vi "create_new_dataset.vi"(8 "error in (no error)":errorcluster, 9 "Variant":variant, 10 "Path":string, 11 "pcfs_hdf5_log in":refnum<class "pcfs_hdf5_log.lvclass">) -> (0 "error out":errorcluster, 3 "pcfs_hdf5_log out":refnum<class "pcfs_hdf5_log.lvclass">)   [LabVIEW 2015, in "pcfs_hdf5_log.lvclass"]
uses:
  pcfs_hdf5_log.lvclass
  pcfs_hdf5_log.lvclass/pcfs_hdf5_log.ctl
  <vilib>/UPVI/lvhdf5/property.llb/LVH5PClassId.ctl
  <vilib>/UPVI/lvhdf5/dataset.llb/LVH5D Operation.ctl
  Detector_Class/Picoquant/Hydraharp/hydraharp_panel/hpanel_acq_modes.ctl
  <vilib>/UPVI/lvhdf5/library.llb/HDF5 Ref.ctl
  <vilib>/UPVI/lvhdf5/group.llb/OpenCreateGroup (String).vi
  <vilib>/UPVI/lvhdf5/datatype.llb/LVH5Tcreate_dataset_type (Variant).vi
  <vilib>/UPVI/lvhdf5/datatype.llb/LVH5Tcreate_dataset_type.xnode
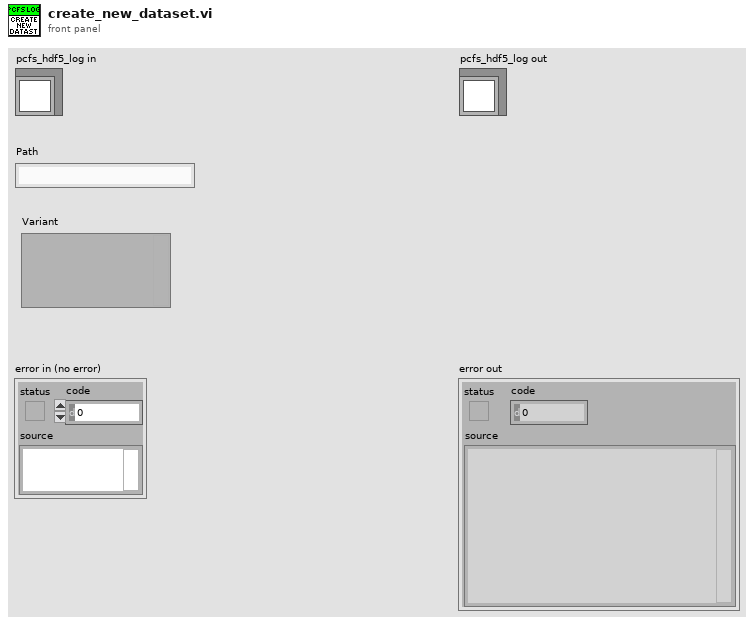
[diagram p1: front panel]
types:
  T1 = typedef "LVH5D Operation.ctl" = enum16{"open", "replace", "create", "open or create", "create or replace", "create or replace with confirmation"}
  T2 = typedef "LVH5PClassId.ctl" = enum32{"H5P_ROOT", "H5P_OBJECT_CREATE", "H5P_FILE_CREATE", "H5P_FILE_ACCESS", "H5P_DATASET_CREATE", "H5P_DATASET_ACCESS", "H5P_DATASET_XFER", "H5P_FILE_MOUNT", "H5P_GROUP_CREATE", "H5P_GROUP_ACCESS", "H5P_DATATYPE_CREATE", "H5P_DATATYPE_ACCESS", "H5P_STRING_CREATE", "H5P_ATTRIBUTE_CREATE", "H5P_OBJECT_COPY", "H5P_LINK_CREATE", "H5P_LINK_ACCESS"}
  T3 = typedef "HDF5 Ref.ctl" = refnum<k1>
  T4 = typedef "hpanel_acq_modes.ctl" = u16
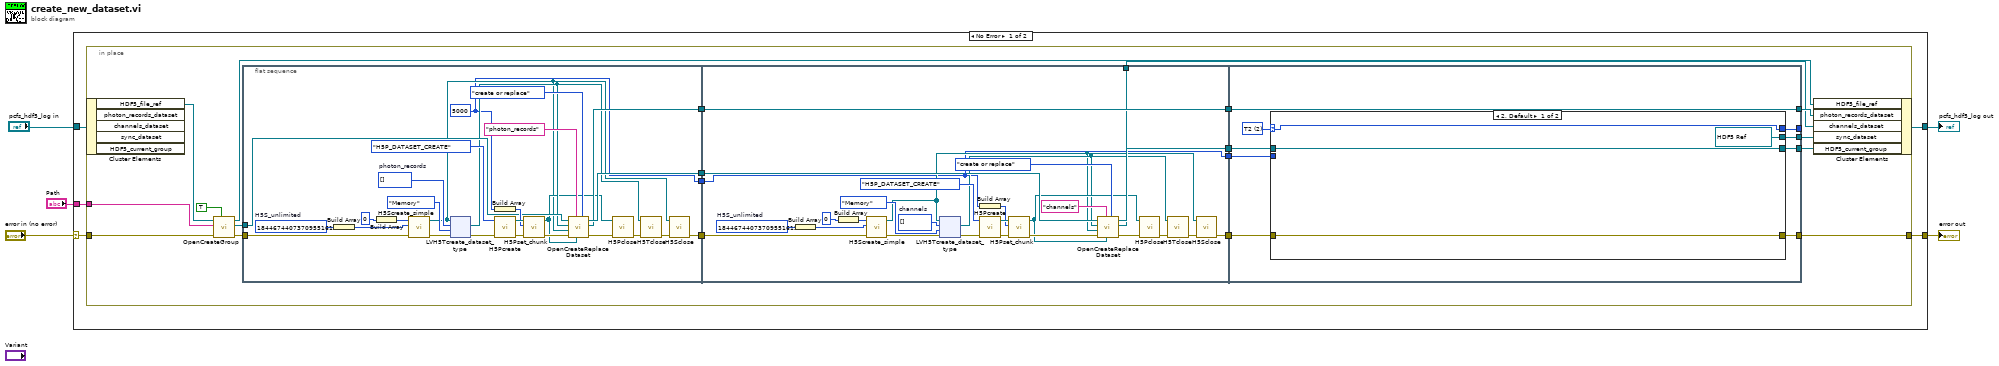
[diagram p0: block diagram]
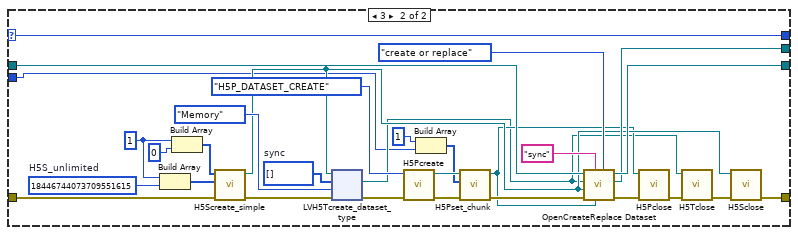
[diagram p2: hidden frame]
diagram:
  n1 = case shown="No Error" "error in (no error)" {
    selector: "error in (no error)" -> [w8 w201]
    tunnel: "pcfs_hdf5_log in" -> [w10 w202]
    tunnel: "Path" -> [w9 _]
    tunnel: [w7 w202] -> w2
    tunnel: [w6 w201] -> w1
    frame No Error {
      n2 = in-place {
        in-place-border: w9 -> [w19]
        in-place-border: w8 -> [w21]
        in-place-border: [w24] -> w6
        n3 = in-place-cluster #1(w10) -> ("HDF5_file_ref"=w17:T3)  [unwired: 4 out]
        n4 = call-poly <vilib>:"OpenCreateGroup.vi"("Create if not found (F)"=TRUE, "error in (no error)"=w21, "Group"=w19, "HDF5 Ref"=w17) -> ("error out"=w20:errorcluster, "HDF5 Group Ref"=w16:T3, "HDF5 Ref out"=w14:T3)  [unwired: 5 in]
        n5 = flat-sequence {
          tunnel: w20 -> [w44]
          tunnel: [w43] -> w29
          tunnel: [w41] -> w28
          tunnel: w16 -> [w40]
          tunnel: [w35] -> w13
          tunnel: [w31] -> w12
          tunnel: w29 -> [w97]
          tunnel: w28 -> [w109]
          tunnel: [w96] -> w27
          tunnel: [w109] -> w26
          tunnel: [w87] -> w25
          tunnel: [w95] -> w23
          tunnel: w13 -> [w98]
          tunnel: w12 -> [w86]
          tunnel: [w86] -> w11
          tunnel: [w142] -> w30
          tunnel: [w138] -> w15
          tunnel: w27 -> [w139]
          tunnel: w26 -> [w142]
          tunnel: w25 -> [w141]
          tunnel: [w140] -> w24
          tunnel: [w137] -> w22
          tunnel: [w136] -> _
          tunnel: w11 -> [w135]
          frame #0 {
            w31 = 5000
            w48 = u64[] []  # photon_records
            w52 = u64 18446744073709551615  # H5S_unlimited
            n6 = Build Array(w52) -> (w51:u64[])
            n7 = Build Array(u64 0 ("element")) -> (w49:u64[])
            n8 = call <vilib>:"H5Screate_simple.vi"("error in (no error)"=w44, "Maximum Dimensions (unlimited)"=w51, "Dimensions"=w49) -> ("error out"=w57:errorcluster, "HDF5 Ref out"=w32:T3)  [unwired: 5 in]
            n9 = xnode "LVH5Tcreate_dataset_type"("HDF5 Location Ref"=w32, "Type"=enum16{"File", "Memory"}."Memory", "error in (no error)"=w57, "Data"=w48) -> ("HDF5 Type Ref"=w34:T3, "error out"=w54:errorcluster)  [unwired: 2 in, 3 out]
            n10 = Build Array(w31) -> (w45:i32[])
            n11 = call <vilib>:"H5Pcreate.vi"("error in (no error)"=w54, "Property List Class"=LVH5PClassId."H5P_DATASET_CREATE") -> ("error out"=w55:errorcluster, "HDF5 Property List Ref"=w56:T3)  [unwired: 6 in]
            n12 = call <vilib>:"H5Pset_chunk.vi"("error in (no error)"=w55, "Dimensions"=w45, "HDF5 Property Ref"=w56) -> ("error out"=w53:errorcluster, "HDF5 Ref out"=w33:T3)  [unwired: 5 in]
            n13 = call <vilib>:"OpenCreateReplace Dataset.vi"("operation (open or create)"=LVH5D_Operation."create or replace", "HDF5 Property List Ref"=w33, "Dataset Path"="photon_records" ("string"), "error in (no error)"=w53, "HDF5 Dataspace Ref"=w32, "HDF5 Datatype Ref"=w34, "HDF5 Ref"=w40) -> ("error out"=w36:errorcluster, "HDF5 Dataset Ref"=w41:T3, "HDF5 Ref out"=w43:T3)  [unwired: 2 in]
            n14 = call <vilib>:"H5Pclose.vi"("error in (no error)"=w36, "HDF5 Property Ref"=w33) -> ("error out"=w38:errorcluster)  [unwired: 7 in]
            n15 = call <vilib>:"H5Tclose.vi"("error in (no error)"=w38, "HDF5 Datatype Ref"=w34) -> ("error out"=w37:errorcluster)  [unwired: 7 in]
            n16 = call <vilib>:"H5Sclose.vi"("error in (no error)"=w37, "HDF5 Dataspace Ref"=w32) -> ("error out"=w35:errorcluster)  [unwired: 7 in]
          }
          frame #1 {
            w85 = u64 18446744073709551615  # H5S_unlimited
            w103 = u8[] []  # channels
            n17 = Build Array(w85) -> (w83:u64[])
            n18 = Build Array(u64 0 ("element")) -> (w82:u64[])
            n19 = call <vilib>:"H5Screate_simple.vi"("error in (no error)"=w98, "Maximum Dimensions (unlimited)"=w83, "Dimensions"=w82) -> ("error out"=w108:errorcluster, "HDF5 Ref out"=w88:T3)  [unwired: 5 in]
            n20 = xnode "LVH5Tcreate_dataset_type"("HDF5 Location Ref"=w88, "Type"=enum16{"File", "Memory"}."Memory", "error in (no error)"=w108, "Data"=w103) -> ("HDF5 Type Ref"=w89:T3, "error out"=w105:errorcluster)  [unwired: 2 in, 3 out]
            n21 = Build Array(w86) -> (w100:i32[])
            n22 = call <vilib>:"H5Pcreate.vi"("error in (no error)"=w105, "Property List Class"=LVH5PClassId."H5P_DATASET_CREATE") -> ("error out"=w106:errorcluster, "HDF5 Property List Ref"=w107:T3)  [unwired: 6 in]
            n23 = call <vilib>:"H5Pset_chunk.vi"("error in (no error)"=w106, "Dimensions"=w100, "HDF5 Property Ref"=w107) -> ("error out"=w104:errorcluster, "HDF5 Ref out"=w90:T3)  [unwired: 5 in]
            n24 = call <vilib>:"OpenCreateReplace Dataset.vi"("operation (open or create)"=LVH5D_Operation."create or replace", "HDF5 Property List Ref"=w90, "Dataset Path"="channels" ("string"), "error in (no error)"=w104, "HDF5 Dataspace Ref"=w88, "HDF5 Datatype Ref"=w89, "HDF5 Ref"=w97) -> ("error out"=w91:errorcluster, "HDF5 Dataset Ref"=w95:T3, "HDF5 Ref out"=w96:T3)  [unwired: 2 in]
            n25 = call <vilib>:"H5Pclose.vi"("error in (no error)"=w91, "HDF5 Property Ref"=w90) -> ("error out"=w93:errorcluster)  [unwired: 7 in]
            n26 = call <vilib>:"H5Tclose.vi"("error in (no error)"=w93, "HDF5 Datatype Ref"=w89) -> ("error out"=w92:errorcluster)  [unwired: 7 in]
            n27 = call <vilib>:"H5Sclose.vi"("error in (no error)"=w92, "HDF5 Dataspace Ref"=w88) -> ("error out"=w87:errorcluster)  [unwired: 7 in]
          }
          frame #2 {
            w134 = T4 2 items=["T2"=2, "T3"=3] ("Mode")
            n28 = case shown="2, Default" w134 {
              selector: w134 -> [w143 w156]
              tunnel: w141 -> [w146 w160]
              tunnel: [w146 w151] -> w140
              tunnel: w139 -> [w145 w159]
              tunnel: [w145 w158] -> w138
              tunnel: [w144 w157] -> w137
              tunnel: [w143 w156] -> w136
              tunnel: w135 -> [_ w147]
              frame 2, Default {
                w144 = T3 refnum items=["HDF5 Ref"] ("HDF5 Dataset Ref")
              }
              frame 3 {
                w166 = u64[] []  # sync
                w169 = u64 1 ("element")
                w171 = u64 18446744073709551615  # H5S_unlimited
                n29 = Build Array(w169, w171) -> (w170:u64[])
                n30 = Build Array(w169, u64 0 ("element")) -> (w167:u64[])
                n31 = call <vilib>:"H5Screate_simple.vi"("error in (no error)"=w160, "Maximum Dimensions (unlimited)"=w170, "Dimensions"=w167) -> ("error out"=w176:errorcluster, "HDF5 Ref out"=w150:T3)  [unwired: 5 in]
                n32 = xnode "LVH5Tcreate_dataset_type"("HDF5 Location Ref"=w150, "Type"=enum16{"File", "Memory"}."Memory", "error in (no error)"=w176, "Data"=w166) -> ("HDF5 Type Ref"=w148:T3, "error out"=w173:errorcluster)  [unwired: 2 in, 3 out]
                n33 = call <vilib>:"H5Pcreate.vi"("error in (no error)"=w173, "Property List Class"=LVH5PClassId."H5P_DATASET_CREATE") -> ("error out"=w174:errorcluster, "HDF5 Property List Ref"=w175:T3)  [unwired: 6 in]
                n34 = Build Array(1 ("element"), w147) -> (w162:i32[])
                n35 = call <vilib>:"H5Pset_chunk.vi"("error in (no error)"=w174, "Dimensions"=w162, "HDF5 Property Ref"=w175) -> ("error out"=w172:errorcluster, "HDF5 Ref out"=w149:T3)  [unwired: 5 in]
                n36 = call <vilib>:"OpenCreateReplace Dataset.vi"("operation (open or create)"=LVH5D_Operation."create or replace", "HDF5 Property List Ref"=w149, "Dataset Path"="sync" ("string"), "error in (no error)"=w172, "HDF5 Dataspace Ref"=w150, "HDF5 Datatype Ref"=w148, "HDF5 Ref"=w159) -> ("error out"=w152:errorcluster, "HDF5 Dataset Ref"=w157:T3, "HDF5 Ref out"=w158:T3)  [unwired: 2 in]
                n37 = call <vilib>:"H5Pclose.vi"("error in (no error)"=w152, "HDF5 Property Ref"=w149) -> ("error out"=w154:errorcluster)  [unwired: 7 in]
                n38 = call <vilib>:"H5Tclose.vi"("error in (no error)"=w154, "HDF5 Datatype Ref"=w148) -> ("error out"=w153:errorcluster)  [unwired: 7 in]
                n39 = call <vilib>:"H5Sclose.vi"("error in (no error)"=w153, "HDF5 Dataspace Ref"=w150) -> ("error out"=w151:errorcluster)  [unwired: 7 in]
              }
            }
          }
        }
        n40 = in-place-cluster #1("HDF5_file_ref"=w14, "photon_records_dataset"=w30, "channels_dataset"=w23, "sync_dataset"=w22, "HDF5_current_group"=w15) -> (w7:refnum<class "pcfs_hdf5_log.lvclass">)
      }
    }
    frame Error {
    }
  }
  "error out" <- w1
  "pcfs_hdf5_log out" <- w2
